vi "Preview Project.vi"(8 "error in (no error)":errorcluster, 11 "Project Model in":refnum<class "Project Model.lvclass">) -> (0 "error out":errorcluster, 3 "Project Model out":refnum<class "Project Model.lvclass">)   [LabVIEW 2013, in "Project Model.lvlib" / "Project Model.lvclass"]
uses:
  Project Model.lvclass
  Project Model.lvclass/Project Model.ctl
  <vilib>/xml/Load XML File.vi
  <vilib>/xml/Close Reference(Node).vi
  Common/File IO/File IO.lvlib
  <vilib>/xml/NI_XML.lvlib
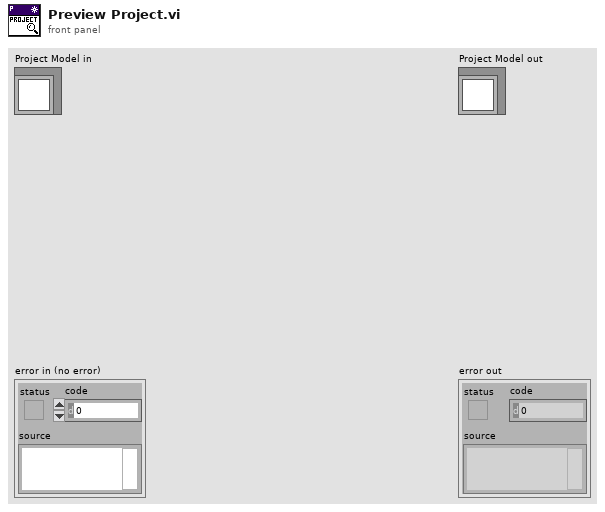
[diagram p1: front panel]
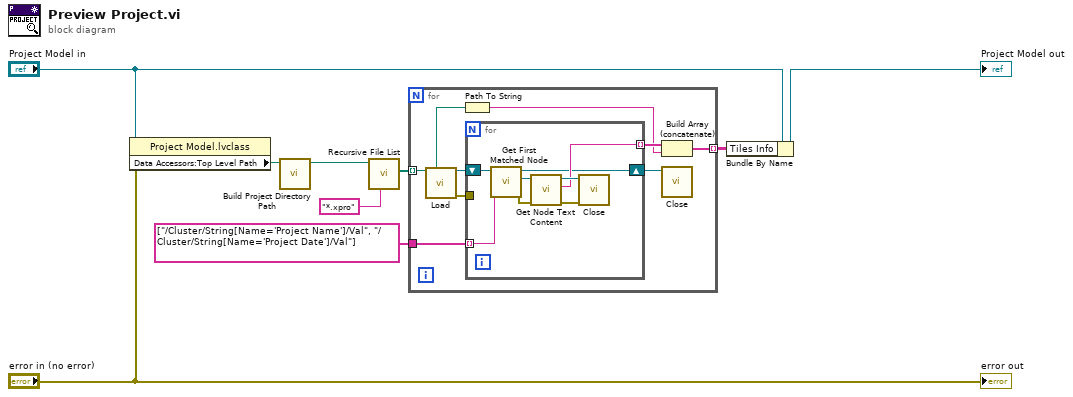
[diagram p0: block diagram]
diagram:
  n1 = property class="Project Model.lvclass"(reference="Project Model in", error in="error in (no error)") -> ("Data Accessors:Top Level Path"=w9:path)  [unwired: 2 out]
  n2 = call "Build Project Directory Path.vi"("Top Level Path"=w9) -> ("Project Directory Path"=w7:path)  [unwired: 10 in]
  n3 = call <vilib>:"Recursive File List.vi"("pattern"="*.xpro", "Folder Path"=w7) -> ("All Files in Dir"=w6:path[])  [unwired: 5 in, 4 out]
  n4 = for {
    tunnel: w6 -> [w14] mode=indexing
    tunnel: string[] ["/Cluster/String[Name='Project Name']/Val", "/Cluster/String[Name='Project Date']/Val"] -> [w16]
    tunnel: [w11] -> w3 mode=indexing
    n5 = call-poly <vilib>:"Load.vi"("path to XML document"=w14) -> ("DOM document out"=w17:refnum<k20>, "error out"=w10:errorcluster)  [unwired: 12 in, 1 out]
    n6 = Path To String(path=w14) -> (string=w13:string)
    n7 = for {
      shift-right: [w18] -> w12
      shift-left: w17 -> [w25]
      tunnel: w16 -> [w24] mode=indexing
      tunnel: [w21] -> w15 mode=indexing
      tunnel: w10 -> [_]
      n8 = call <vilib>:"Get First Matched Node.vi"("XPath expression"=w24, "node in"=w25) -> ("error out"=w19:errorcluster, "node result"=w23:refnum<k20>, "node out"=w18:refnum<k20>)  [unwired: 7 in]
      n9 = call <vilib>:"Get Node Text Content.vi"("error in (no error)"=w19, "node in"=w23) -> ("error out"=w20:errorcluster, "node text"=w21:string, "node out"=w22:refnum<k20>)  [unwired: 7 in]
      n10 = call-poly <vilib>:"Close.vi"("error in (no error)"=w20, "node"=w22) -> ()  [unwired: 7 in, 1 out]
    }
    n11 = Build Array (concatenate)(w15, w13) -> (w11:string[])
    n12 = call-poly <vilib>:"Close.vi"("node"=w12) -> ()  [unwired: 8 in, 1 out]
  }
  n13 = Bundle By Name(cluster="Project Model in", "Tiles Info"=w3) -> (→"Project Model out":refnum<class "Project Model.lvclass">)
  "error out" <- "error in (no error)"
